vi "Set Setpoint Source.vi"(7 "listen period":sgl=0.1, 8 "error in":errorcluster, 10 "setpoint source":u8(ring)=3 caption="Setpoint Source (Write)" items=["Undefined", "0..5 volt or 0..20mA input", "1..5 volt or 4..20mA input", "Communication input"], 11 "Brooks MFC in":refnum<class "Brooks MFC.lvclass">) -> (0 "error out":errorcluster, 2 "setpoint source":u8(ring)=3 caption="Setpoint Source (Read)" items=["Undefined", "0..5 volt or 0..20mA input", "1..5 volt or 4..20mA input", "Communication input"], 3 "Brooks MFC out":refnum<class "Brooks MFC.lvclass">)   [LabVIEW 2016, in "Brooks MFC.lvclass"]
uses:
  Brooks MFC.lvclass
  Brooks MFC.lvclass/Brooks MFC.ctl
  Instance           3 30Saved   Select Setpoint Source .vi
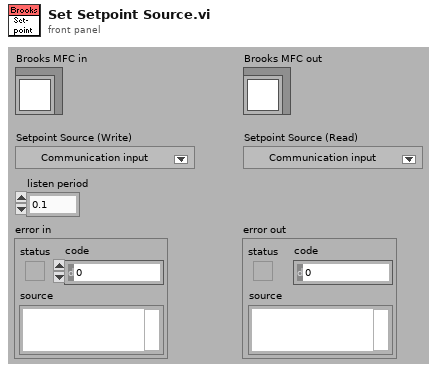
[diagram p1: front panel]
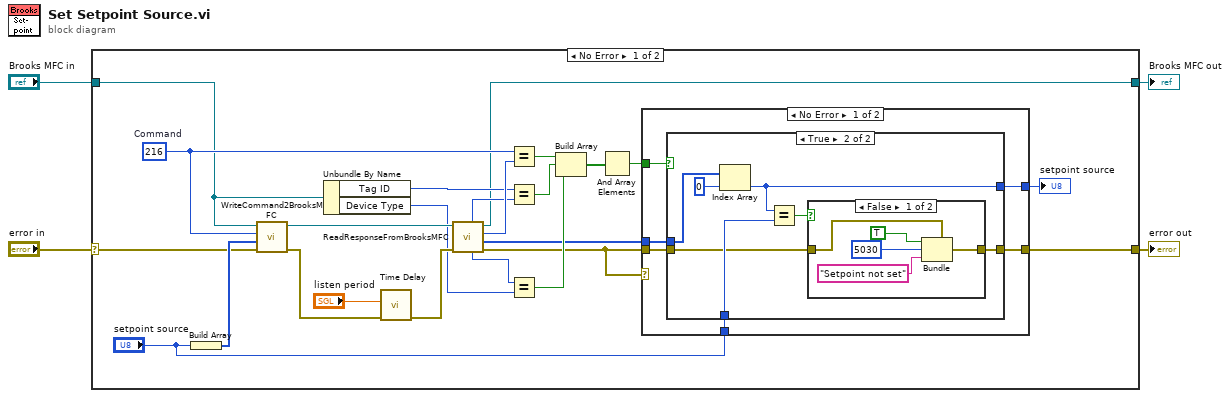
[diagram p0: block diagram]
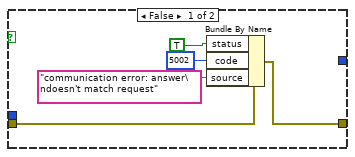
[diagram p2: hidden frame]
diagram:
  n1 = case shown="No Error" "error in" {
    selector: "error in" -> [w8 w54]
    tunnel: "Brooks MFC in" -> [w14 w55]
    tunnel: [w6 w54] -> w2
    tunnel: [w5 w55] -> w1
    frame No Error {
      w15 = u8 216  # Command
      n2 = Build Array("setpoint source") -> (w16:u8[])
      n3 = call "WriteCommand2BrooksMFC.vi"("error in"=w8, "Data"=w16, "Command"=w15, "Brooks MFC in"=w14) -> ("error out"=w27:errorcluster, "Brooks MFC out"=w9:refnum<class "Brooks MFC.lvclass">)  [unwired: 5 in, 1 out]
      n4 = Unbundle By Name(w14) -> ("Tag ID"=w13:u32, "Device Type"=w7:u8)
      n5 = call "Time Delay"("error in (no error)"=w27, "Delay Time (s)"="listen period") -> ("error out"=w26:errorcluster)  [unwired: 9 in]
      n6 = call "ReadResponseFromBrooksMFC.vi"("error in"=w26, "Brooks MFC in"=w9) -> ("error out"=w11:errorcluster, "Data"=w10:u8[], "Command"=w28:u8, "Brooks MFC out"=w5:refnum<class "Brooks MFC.lvclass">, "device type"=w23:u8, "tag ID"=w24:u32)  [unwired: 4 in]
      n7 = Equal?(x=w15, y=w28) -> (x = y?=w22:bool)
      n8 = Equal?(x=w13, y=w24) -> (x = y?=w19:bool)
      n9 = Equal?(x=w23, y=w7) -> (x = y?=w18:bool)
      n10 = Build Array(w22, w19, w18) -> (w21:bool[])
      n11 = And Array Elements(Boolean array=w21) -> (logical AND=w20:bool)
      n12 = case shown="No Error" w11 {
        tunnel: w11 -> [w34 w53]
        tunnel: w10 -> [w33 _]
        tunnel: [w32 w53] -> w6
        tunnel: w20 -> [w31 _]
        tunnel: [w30 _] -> w17
        tunnel: "setpoint source" -> [w29 _]
        frame No Error {
          n13 = case shown="True" w31 {
            tunnel: w33 -> [_ w46]
            tunnel: w34 -> [w37 w40]
            tunnel: [w36 w41] -> w32
            tunnel: [_ w43] -> w30
            tunnel: w29 -> [_ w42]
            frame False {
              n14 = Bundle By Name(cluster=w37, "status"=TRUE ("Bundle Element"), "code"=5002 ("Bundle Element"), "source"="communication error: answer\ndoesn't match request") -> (w36:errorcluster)
            }
            frame True {
              n15 = Index Array(array=w46, index=0 ("Index")) -> (element=w43:u8)
              n16 = Equal?(x=w43, y=w42) -> (x = y?=w44:bool)
              n17 = case shown="False" w44 {
                tunnel: [w47 w52] -> w41
                tunnel: w40 -> [w51 w52]
                frame False {
                  n18 = Bundle(cluster=w51, "status"=TRUE, "code"=5030, "source"="Setpoint not set") -> (w47:errorcluster)
                }
                frame True {
                }
              }
            }
          }
        }
        frame Error {
        }
      }
      "setpoint source" <- w17
    }
    frame Error {
    }
  }
  "error out" <- w2
  "Brooks MFC out" <- w1
